vi "Ref_Num_Set_Header.vi"(0 "Report Array Header":refnum<vi>, 1 "Test Fixture (OUTPUT)":refnum<vi>, 2 "Frequency":refnum<vi>, 3 "Test Type (OUTPUT)":refnum<vi>, 4 "AddTestComment":string, 5 "Test Level value":refnum<vi>, 6 "Current LCR Voltage":refnum<vi>, 8 "Operator":refnum<vi>, 9 "SHORT Compensation":refnum<vi>, 12 "Request Number":refnum<vi>, 13 "OPEN Compensation":refnum<vi>, 14 "Date (DD/MM/YYYY)":refnum<vi>, 15 "Calibration Short : Started":refnum<vi>, 16 "Captest?":refnum<vi>, 17 "Open Calibration : Started":refnum<vi>, 20 "Lot Date":refnum<vi>, 21 "Part Number":refnum<vi>, 23 "Test System":refnum<vi>, 24 "Lot Number":refnum<vi>, 25 "Test Comments":refnum<vi>, 27 "Stop":refnum<vi>) -> ()   [LabVIEW 2020]
uses:
  Global 1.vi
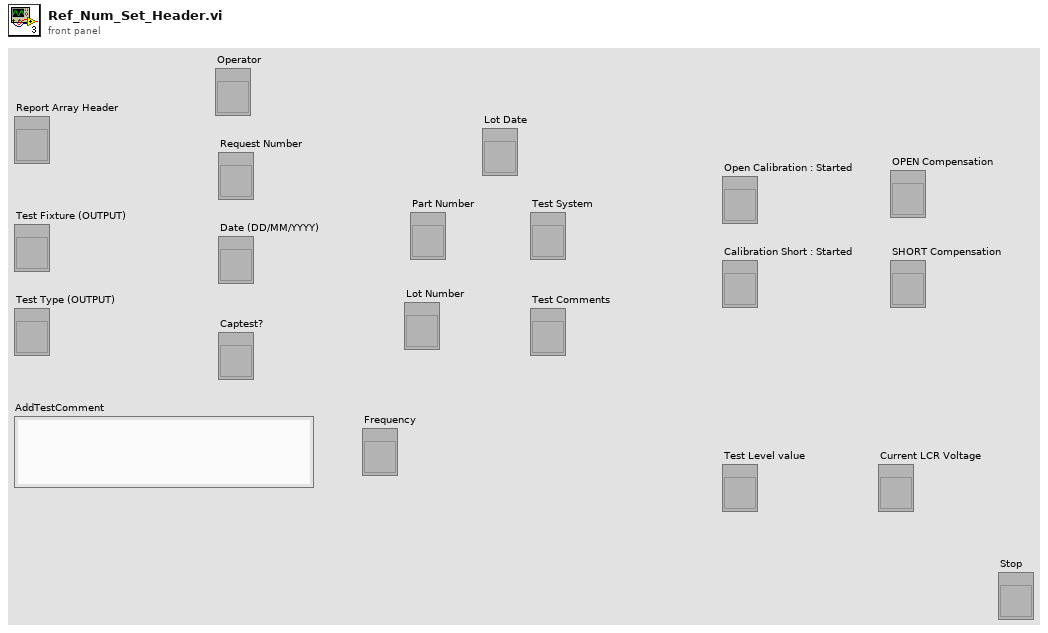
[diagram p1: front panel]
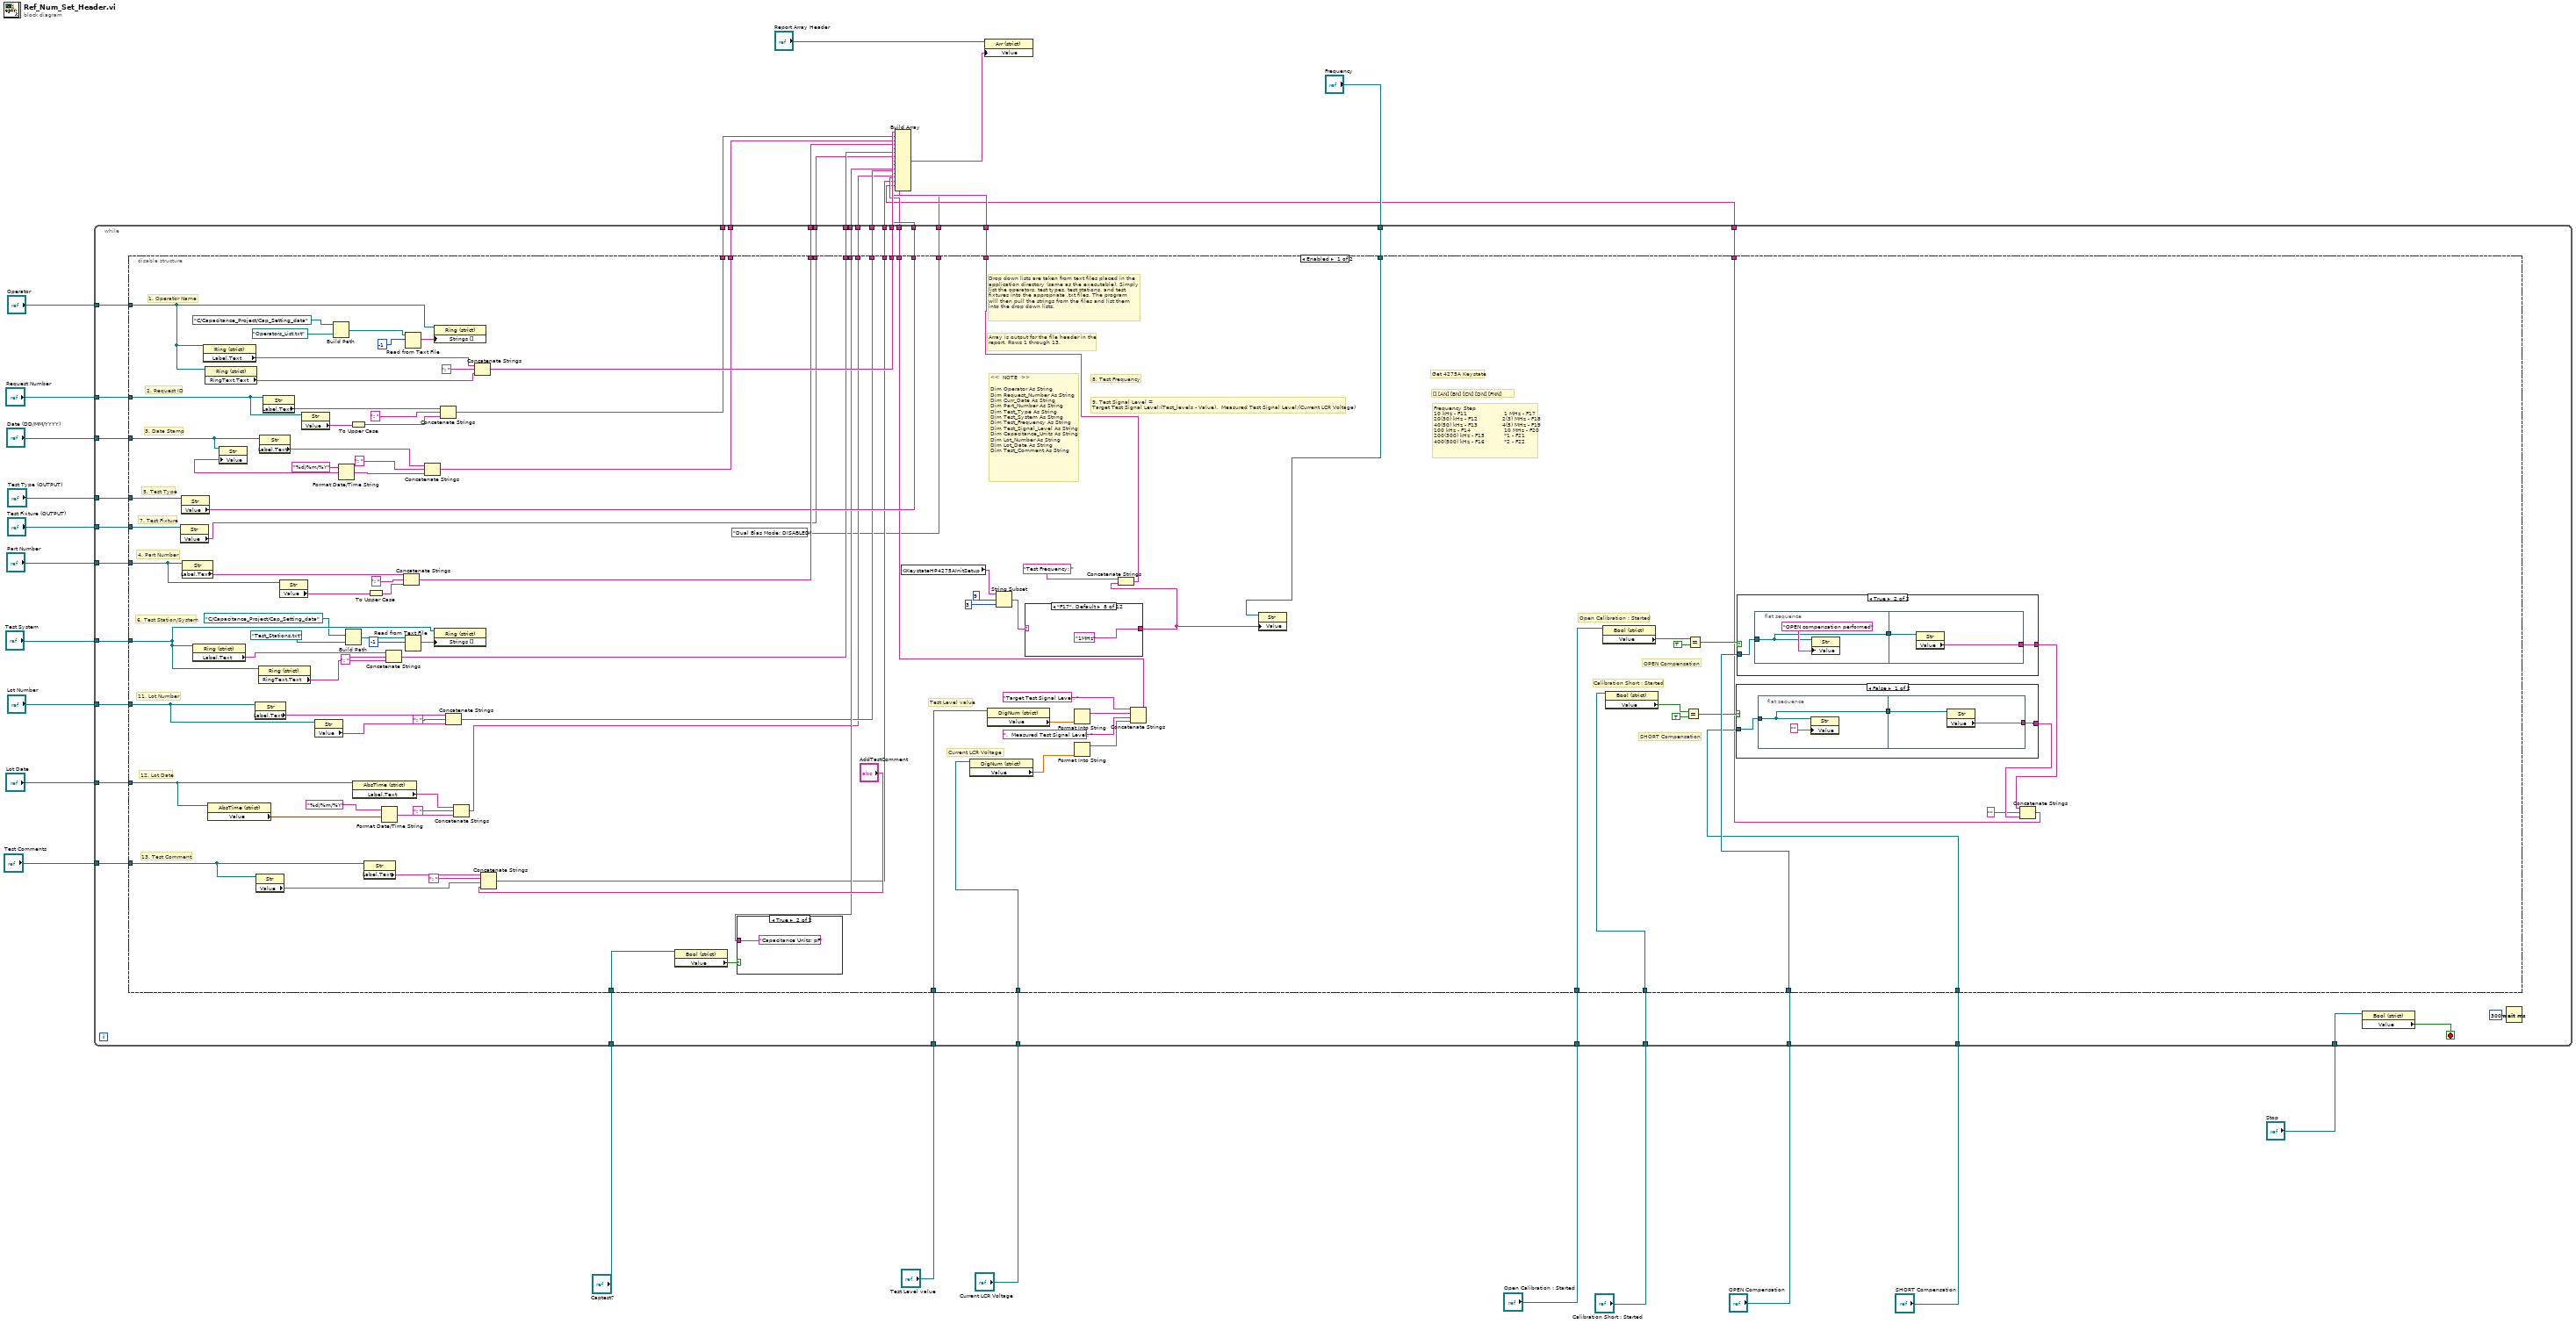
[diagram p0: block diagram]
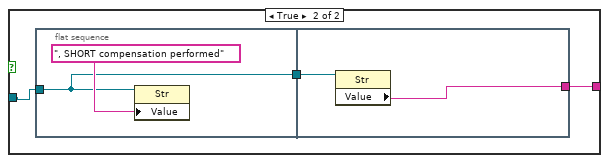
[diagram p2: hidden frame]
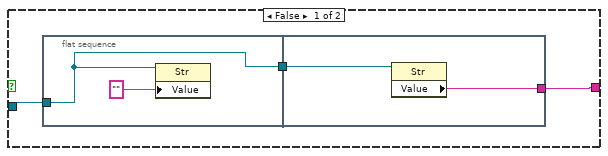
[diagram p3: hidden frame]
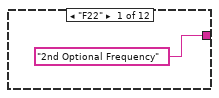
[diagram p4: hidden frame]
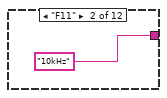
[diagram p5: hidden frame]
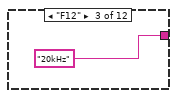
[diagram p6: hidden frame]
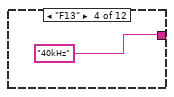
[diagram p7: hidden frame]
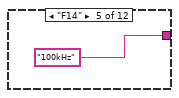
[diagram p8: hidden frame]
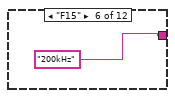
[diagram p9: hidden frame]
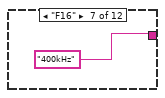
[diagram p10: hidden frame]
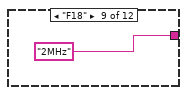
[diagram p11: hidden frame]
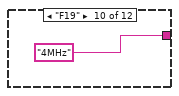
[diagram p12: hidden frame]
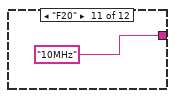
[diagram p13: hidden frame]
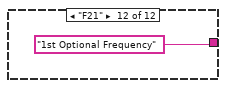
[diagram p14: hidden frame]
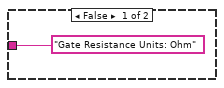
[diagram p15: hidden frame]
diagram:
  n1 = while {
    tunnel: "Operator" -> [w72]
    tunnel: "Request Number" -> [w71]
    tunnel: "Test Type (OUTPUT)" -> [w70]
    tunnel: "Test Fixture (OUTPUT)" -> [w69]
    tunnel: "Part Number" -> [w68]
    tunnel: "Test System" -> [w67]
    tunnel: "Lot Number" -> [w66]
    tunnel: "Lot Date" -> [w65]
    tunnel: "Test Comments" -> [w64]
    tunnel: "Captest?" -> [w63]
    tunnel: "Test Level value" -> [w62]
    tunnel: "Current LCR Voltage" -> [w61]
    tunnel: "Open Calibration : Started" -> [w60]
    tunnel: "Calibration Short : Started" -> [w59]
    tunnel: "OPEN Compensation" -> [w58]
    tunnel: "SHORT Compensation" -> [w57]
    tunnel: "Date (DD/MM/YYYY)" -> [w56]
    tunnel: "Frequency" -> [w55]
    tunnel: [w54] -> w17
    tunnel: [w53] -> w16
    tunnel: [w52] -> w15
    tunnel: [w51] -> w14
    tunnel: [w50] -> w13
    tunnel: [w49] -> w12
    tunnel: [w48] -> w11
    tunnel: [w47] -> w10
    tunnel: [w46] -> w9
    tunnel: [w45] -> w8
    tunnel: [w44] -> w7
    tunnel: [w43] -> w6
    tunnel: [w42] -> w5
    tunnel: [w41] -> w4
    tunnel: [w40] -> w3
    tunnel: "Stop" -> [w37]
    stop <- w38 stop-if-true
    n2 = disable-structure shown="Enabled" {
      disable-tunnel: w72 -> [w142 _]
      disable-tunnel: w71 -> [w139 _]
      disable-tunnel: w56 -> [w138 _]
      disable-tunnel: w70 -> [w135 _]
      disable-tunnel: w69 -> [w134 _]
      disable-tunnel: w68 -> [w132 _]
      disable-tunnel: w67 -> [w130 _]
      disable-tunnel: w66 -> [w128 _]
      disable-tunnel: w65 -> [w125 _]
      disable-tunnel: w64 -> [w122 _]
      disable-tunnel: w63 -> [w120 _]
      disable-tunnel: w62 -> [w119 _]
      disable-tunnel: w61 -> [w118 _]
      disable-tunnel: w60 -> [w117 _]
      disable-tunnel: w59 -> [w116 _]
      disable-tunnel: w58 -> [w115 _]
      disable-tunnel: w57 -> [w114 _]
      disable-tunnel: w55 -> [w113 _]
      disable-tunnel: [w87 _] -> w54
      disable-tunnel: [w86 _] -> w53
      disable-tunnel: [w85 _] -> w52
      disable-tunnel: [w84 _] -> w51
      disable-tunnel: [w83 _] -> w50
      disable-tunnel: [w82 _] -> w49
      disable-tunnel: [w81 _] -> w48
      disable-tunnel: [w80 _] -> w47
      disable-tunnel: [w79 _] -> w46
      disable-tunnel: [w78 _] -> w45
      disable-tunnel: [w77 _] -> w44
      disable-tunnel: [w76 _] -> w43
      disable-tunnel: [w75 _] -> w42
      disable-tunnel: [w74 _] -> w41
      disable-tunnel: ["Dual Bias Mode: DISABLED" ("element") _] -> w40
      frame Enabled {
        # "SHORT Compensation"
        # "OPEN Compensation"
        # "Calibration Short : Started"
        # "Open Calibration : Started"
        # "Current LCR Voltage"
        # "Test Level value"
        # "7. Test Fixture"
        # "Frequency Step\n10 kHz - F11                     1 MHz - F17\n20(30) kHz - F12              2(3) MHz - F18\n40(50) kHz - F13              4(5) MHz - F19\n100 kHz - F14                   10 MHz - F20\n200(300) kHz - F15           *1 - F21\n400(500) kHz - F16           *2 - F22"
        # "[] [AN] [BN] [CN] [DN] [FNN]"
        # "Get 4275A Keystate"
        # "8. Test Frequency"
        # "<<  NOTE  >>\n\nDim Operator As String\nDim Request_Number As String\nDim Curr_Date As String\nDim Part_Number As String\nDim Test_Type As String\nDim Test_System As String\nDim Test_Frequency As String\nDim Test_Signal_Level As String\nDim Capacitance_Units As String\nDim Lot_Number As String\nDim Lot_Date As String\nDim Test_Comment As String"
        # "13. Test Comment"
        # "Array is output for the file header in the \nreport. Rows 1 through 13."
        # "Drop down lists are taken from text files placed in the \napplication directory (same as the executable). Simply\nlist the operators, test types, test stations, and test\nfixtures into the appropriate .txt files. The program\nwill then pull the strings from the files and list them\ninto the drop down lists."
        # "12. Lot Date"
        # "11. Lot Number"
        # "9. Test Signal Level = \nTarget Test Signal Level:(Test_levels - Value),  Measured Test Signal Level:(Current LCR Voltage)"
        # "6. Test Station/System"
        # "5. Test Type"
        # "4. Part Number"
        # "3. Date Stamp"
        # "2. Request ID"
        # "1. Operator Name"
        n3 = property class="Str"(reference=w134) -> ("Value"=w81:string)  [unwired: 1 in, 2 out]
        n4 = property class="Str"(reference=w135) -> ("Value"=w83:string)  [unwired: 1 in, 2 out]
        n5 = property class="Str"(reference=w132) -> ("Label.Text"=w133:string)  [unwired: 1 in, 2 out]
        n6 = property on="Property Node" class="Ring (strict)"(reference=w130) -> ("Label.Text"=w90:string)  [unwired: 1 in, 2 out]
        n7 = property on="Property Node" class="Ring (strict)"(reference=w142) -> ("Label.Text"=w151:string)  [unwired: 1 in, 2 out]
        n8 = property on="Property Node" class="Ring (strict)"(reference=w142) -> ("RingText.Text"=w165:string)  [unwired: 1 in, 2 out]
        n9 = property class="AbsTime (strict)"(reference=w125) -> ("Value"=w124:timestamp)  [unwired: 1 in, 2 out]
        n10 = property class="Str"(reference=w128) -> ("Label.Text"=w129:string)  [unwired: 1 in, 2 out]
        n11 = property class="Str"(reference=w122) -> ("Value"=w121:string)  [unwired: 1 in, 2 out]
        n12 = property on="Property Node" class="Ring (strict)"(reference=w130) -> ("RingText.Text"=w149:string)  [unwired: 1 in, 2 out]
        n13 = property class="Str"(reference=w138) -> ("Label.Text"=w136:string)  [unwired: 1 in, 2 out]
        n14 = property class="Str"(reference=w139) -> ("Label.Text"=w141:string)  [unwired: 1 in, 2 out]
        n15 = property class="Str"(reference=w132) -> ("Value"=w131:string)  [unwired: 1 in, 2 out]
        n16 = property class="Str"(reference=w139) -> ("Value"=w140:string)  [unwired: 1 in, 2 out]
        n17 = property class="Str"(reference=w128) -> ("Value"=w127:string)  [unwired: 1 in, 2 out]
        n18 = Build Path(base path=path "C:/Capacitance_Project/Cap_Setting_data", name or relative path=path "Operators_List.txt" ("file (use dialog)")) -> (appended path=w154:path)
        n19 = Format Date/Time String(time format string (%c)="%d/%m/%Y") -> (date/time string=w137:string)  [unwired: 2 in]
        n20 = property class="Str"(reference=w138, "Value"=w137) -> ()  [unwired: 1 in, 2 out]
        n21 = Build Path(base path=path "C:/Capacitance_Project/Cap_Setting_data", name or relative path=path "Test_Stations.txt" ("file (use dialog)")) -> (appended path=w152:path)
        n22 = To Upper Case(1:w140) -> (0:w159:string)
        n23 = property class="AbsTime (strict)"(reference=w125) -> ("Label.Text"=w126:string)  [unwired: 1 in, 2 out]
        n24 = property class="Str"(reference=w122) -> ("Label.Text"=w123:string)  [unwired: 1 in, 2 out]
        n25 = To Upper Case(1:w131) -> (0:w160:string)
        n26 = Format Date/Time String(time format string (%c)="%d/%m/%Y", seconds (now)=w124) -> (date/time string=w146:string)  [unwired: 1 in]
        n27 = Concatenate Strings(w90, ": " ("string"), w149) -> (w82:string)
        n28 = Concatenate Strings(w133, ": " ("string"), w160) -> (w84:string)
        n29 = Read from Text File(file (use dialog)=w154, count=-1) -> (text=w167:string[])  [unwired: 2 in, 3 out]
        n30 = Read from Text File(file (use dialog)=w152, count=-1) -> (text=w157:string[])  [unwired: 2 in, 3 out]
        n31 = Concatenate Strings(w136, ": " ("string"), w137) -> (w85:string)
        n32 = property on="Property Node" class="Ring (strict)"(reference=w142, "Strings []"=w167) -> ()  [unwired: 1 in, 2 out]
        n33 = property on="Property Node" class="Ring (strict)"(reference=w130, "Strings []"=w157) -> ()  [unwired: 1 in, 2 out]
        n34 = Concatenate Strings(w141, ": " ("string"), w159) -> (w86:string)
        n35 = Concatenate Strings(w129, ": " ("string"), w127) -> (w77:string)
        n36 = Concatenate Strings(w126, ": " ("string"), w146) -> (w76:string)
        n37 = Concatenate Strings(w151, ": " ("string"), w165) -> (w87:string)
        n38 = Concatenate Strings(w123, ": " ("string"), w121, "AddTestComment") -> (w75:string)
        n39 = property on="Property Node" class="Bool (strict)"(reference=w120) -> ("Value"=w143:bool)  [unwired: 1 in, 2 out]
        n40 = case shown="True" w143 {
          tunnel: ["Gate Resistance Units: Ohm" ("element") "Capacitance Units: pF" ("element")] -> w78
          frame False {
          }
          frame True {
          }
        }
        n41 = global read "Global 1.vi" "KeystateHP4275AInitSetup"() -> (w103:string)
        n42 = property class="DigNum (strict)"(reference=w118) -> ("Value"=w101:dbl)  [unwired: 1 in, 2 out]
        n43 = property class="DigNum (strict)"(reference=w119) -> ("Value"=w102:dbl)  [unwired: 1 in, 2 out]
        n44 = String Subset(string=w103, offset (0)=9, length (rest)=3 ("length (rest)")) -> (substring=w106:string)
        n45 = case shown="\"F17\", Default" w106 {
          tunnel: ["2nd Optional Frequency" "10kHz" "20kHz" "40kHz" "100kHz" "200kHz" "400kHz" "1MHz" "2MHz" "4MHz" "10MHz" "1st Optional Frequency"] -> w100
          frame "F22" {
          }
          frame "F11" {
          }
          frame "F12" {
          }
          frame "F13" {
          }
          frame "F14" {
          }
          frame "F15" {
          }
          frame "F16" {
          }
          frame "F17", Default {
          }
          frame "F18" {
          }
          frame "F19" {
          }
          frame "F20" {
          }
          frame "F21" {
          }
        }
        n46 = Format Into String(w102) -> (resulting string=w110:string)  [unwired: 3 in, 1 out]
        n47 = Format Into String(w101) -> (resulting string=w108:string)  [unwired: 3 in, 1 out]
        n48 = Concatenate Strings("Test Frequency: " ("string"), w100) -> (w80:string)
        n49 = Concatenate Strings("Target Test Signal Level: " ("string"), w110, ",  Measured Test Signal Level: " ("string"), w108) -> (w79:string)
        n50 = property class="Str"(reference=w113, "Value"=w100) -> ()  [unwired: 1 in, 2 out]
        n51 = property class="Bool (strict)"(reference=w117) -> ("Value"=w92:bool)  [unwired: 1 in, 2 out]
        n52 = property class="Bool (strict)"(reference=w116) -> ("Value"=w91:bool)  [unwired: 1 in, 2 out]
        n53 = Equal?(x=w91, y=TRUE) -> (x = y?=w96:bool)
        n54 = Equal?(x=w92, y=TRUE) -> (x = y?=w97:bool)
        n55 = case shown="False" w96 {
          tunnel: [w170 w177] -> w99
          tunnel: w114 -> [w169 w176]
          frame False {
            n56 = flat-sequence {
              tunnel: w169 -> [w171]
              tunnel: [w171] -> w168
              tunnel: [w174] -> w170
              tunnel: w168 -> [w173]
              frame #0 {
                n57 = property class="Str"(reference=w171, "Value"="" ("OPEN Compensation")) -> ()  [unwired: 1 in, 2 out]
              }
              frame #1 {
                n58 = property class="Str"(reference=w173) -> ("Value"=w174:string)  [unwired: 1 in, 2 out]
              }
            }
          }
          frame True {
            n59 = flat-sequence {
              tunnel: w176 -> [w178]
              tunnel: [w178] -> w175
              tunnel: [w181] -> w177
              tunnel: w175 -> [w180]
              frame #0 {
                n60 = property class="Str"(reference=w178, "Value"=", SHORT compensation performed" ("SHORT Compensation")) -> ()  [unwired: 1 in, 2 out]
              }
              frame #1 {
                n61 = property class="Str"(reference=w180) -> ("Value"=w181:string)  [unwired: 1 in, 2 out]
              }
            }
          }
        }
        n62 = case shown="True" w97 {
          tunnel: [w184 w191] -> w98
          tunnel: w115 -> [w183 w190]
          frame False {
            n63 = flat-sequence {
              tunnel: w183 -> [w185]
              tunnel: [w185] -> w182
              tunnel: [w188] -> w184
              tunnel: w182 -> [w187]
              frame #0 {
                n64 = property class="Str"(reference=w185, "Value"="" ("OPEN Compensation")) -> ()  [unwired: 1 in, 2 out]
              }
              frame #1 {
                n65 = property class="Str"(reference=w187) -> ("Value"=w188:string)  [unwired: 1 in, 2 out]
              }
            }
          }
          frame True {
            n66 = flat-sequence {
              tunnel: w190 -> [w192]
              tunnel: [w192] -> w189
              tunnel: [w195] -> w191
              tunnel: w189 -> [w194]
              frame #0 {
                n67 = property class="Str"(reference=w192, "Value"="OPEN compensation performed" ("OPEN Compensation")) -> ()  [unwired: 1 in, 2 out]
              }
              frame #1 {
                n68 = property class="Str"(reference=w194) -> ("Value"=w195:string)  [unwired: 1 in, 2 out]
              }
            }
          }
        }
        n69 = Concatenate Strings(w98, "" ("string"), w99) -> (w74:string)
      }
      frame Disabled {
      }
    }
    n70 = property class="Bool (strict)"(reference=w37) -> ("Value"=w38:bool)  [unwired: 1 in, 2 out]
    n71 = Wait (ms)(milliseconds to wait=u32 300) -> ()  [unwired: 1 out]
  }
  n72 = Build Array(w17, w16, w15, w14, w13, w12, w11, w10, w9, w8, w7, w6, w5, w4, w3) -> (w2:string[])
  n73 = property class="Arr (strict)"(reference="Report Array Header", "Value"=w2) -> ()  [unwired: 1 in, 2 out]
